vi "oldECG AF SPI Input.vi"() -> ()   [LabVIEW 2013]
uses:
  ECG Data.ctl
  IBP Data.ctl
  Trigger Params.ctl
  Lead Enum.ctl
  <vilib>/Platform/TimedLoop/XDataNode/timing_clust.ctl
  <vilib>/Platform/TimedLoop/XDataNode/nitl_modes.ctl
  <vilib>/Platform/TimedLoop/XDataNode/wakeup.ctl
  Gradient Data.ctl
  All Data.ctl
  <vilib>/rvi/Emulation/niFpgaSctlEmulationGetInTimedLoop.vi
  <vilib>/rvi/Emulation/niFpgaEmulationReportErrorSimple.vi
  <vilib>/rvi/Emulation/niFpgaGetClockAttributes.vi
  <vilib>/rvi/Emulation/niFpgaCriticalErrorInLSC.vi
  <vilib>/rvi/eio/common/nirviEmuTemplateMethod_errors.vi
  <vilib>/rvi/DataTransferAndStorage/Container/Common/niFpgaContainerGetUniqueNameForEmu.vi
  <vilib>/rvi/DataTransferAndStorage/Container/Common/niFpgaContainerSetEmuInfo.vi
  <vilib>/rvi/eio/common/nirviEmuReportErrorAndStop.vi
  <vilib>/rvi/Emulation/niFpgaProcessEmulError.vi
  <vilib>/rvi/Analysis/common/codeGenErrors/XNode/niFpgaXNodeCodeGenErrorHandle.vi
  <vilib>/rvi/DataTransferAndStorage/Container/Common/niFpgaContainerExecOnDevCompGetState.vi
  <vilib>/rvi/FIFO/Fifo_Resource/nirvififoEmulationWriteFpgaImpl.vi
  <vilib>/rvi/interface/RandomDataEmulation/nirviRandomDataFPGAFIFO.vi
  <vilib>/rvi/interface/RandomDataEmulation/niFpgaRandomDataHandleErrors.vi
  <vilib>/rvi/FIFO/Fifo_Resource/nirvififoEmulationGetNumberOfElementsToReadFpgaImpl.vi
  <vilib>/rvi/FIFO/Fifo_Resource/nirvififoEmulationReadFpgaImpl.vi
  <vilib>/Platform/TimedLoop/XDataNode/XDataNode.xnode
  <vilib>/eio/EIONode/EIONode.xnode
  <vilib>/rvi/LocalResourceManager/LocalResourceManager.xnode
  <vilib>/eio/EIOMethodNode/EIOMethodNode.xnode
  <vilib>/rvi/Analysis/measure/butterworth/XNode/niFpgaButterworthFilter.xnode
  <vilib>/rvi/Analysis/measure/LMRsmpl/XNode/niFPGA Rational Resampler.xnode
  <vilib>/rvi/DataTransferAndStorage/Container/XNode/niFpgaContainer.xnode
  <vilib>/rvi/FIFO/Fifo_Resource/niFpgaFifoEmulationRefIn.vi
  <vilib>/Platform/TimedLoop/XDataNode/XDNodeRunTimeDep.lvlib
panel:
  out "LL Out":i16
  out "LA Out":i16
  out "RA Out":i16
  out "LL In":i16
  out "LA In":i16
  out "RA In":i16
  in  "HPF":bool
  in  "Trigger":T1
  out "IBP Data":T3
  out "ECG Data":T4
  in  "stop":bool
  in  "Reset":bool
  out "Send":bool
  out "WeightSum":fxp<+/-,33,19> format="%.20g"
  out "BetaProduct":fxp<+/-,32,-1> format="%.33g"
  out "Loop Time":u32
  in  "Filter Size":i16
  out "I In":i16
  out "II In":i16
  out "III In":i16
  out "aVR In":i16
  out "aVL In":i16
  out "aVF In":i16
  out "V1 In":i16
  out "V2 In":i16
  out "V3 In":i16
  out "V4 In":i16
  out "V5 In":i16
  out "V6 In":i16
  out "V4 Out":i16
  out "V5 Out":i16
  out "V6 Out":i16
  out "IBP3":i16
  out "IBP2":i16
  out "IBP1":i16
  in  "Start 0":bool
  in  "Filter On":bool=TRUE
  in  "Beta":fxp<+/-,32,-16>
  out "V3 Out":i16
  out "V2 Out":i16
  out "V1 Out":i16
  out "aVF Out":i16
  out "aVL Out":i16
  out "aVR Out":i16
  out "III Out":i16
  out "II Out":i16
  out "I Out":i16
  out "V6":i16
  out "V5":i16
  out "V4":i16
  out "V3":i16
  out "V2":i16
  out "V1":i16
  out "LL":i16
  out "LA":i16
  out "Actual Loop Rate (Ticks)":u32
  out "Late? Latched":bool
  out "RA":i16
  in  "Loop Rate (Ticks)":u32=4000
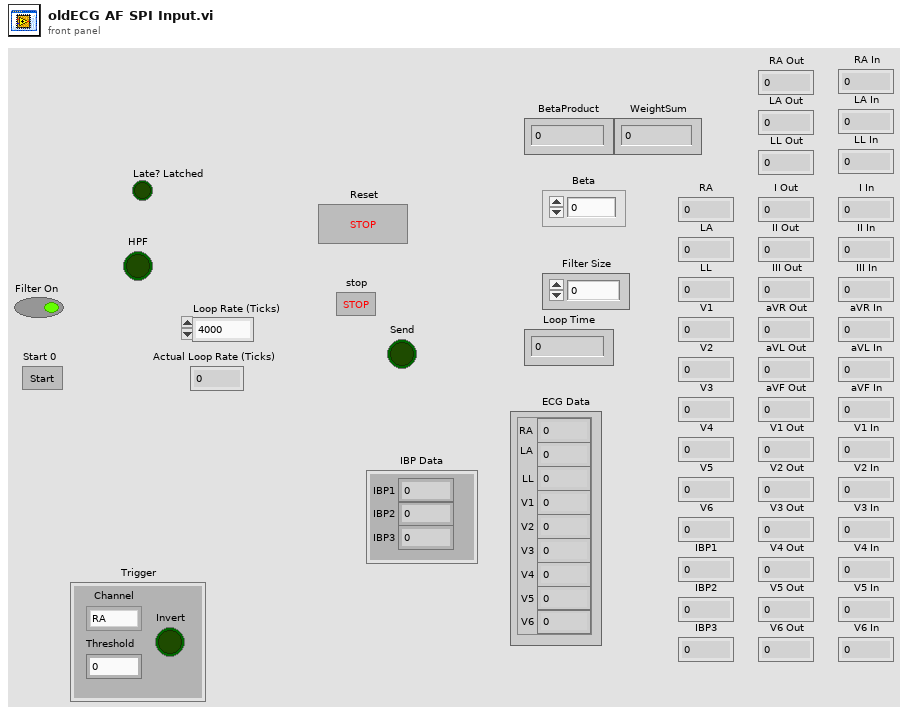
[diagram p1: front panel]
types:
  T1 = typedef "Trigger Params.ctl" = cluster{"Channel":T2, "Threshold":i16, "Invert":bool}
  T2 = typedef "Lead Enum.ctl" = enum16{"RA", "LA", "LL", "V1", "V2", "V3", "V4", "V5", "V6", "I", "II", "III", "aVR", "aVL", "aVF", "Vw"}
  T3 = typedef "IBP Data.ctl" = cluster{"IBP1":fxp<+/-,16,16>, "IBP2":fxp<+/-,16,16>, "IBP3":fxp<+/-,16,16>}
  T4 = typedef "ECG Data.ctl" = cluster{"RA":fxp<+/-,16,16>, "LA":fxp<+/-,16,16>, "LL":fxp<+/-,16,16>, "V1":fxp<+/-,16,16>, "V2":fxp<+/-,16,16>, "V3":fxp<+/-,16,16>, "V4":fxp<+/-,16,16>, "V5":fxp<+/-,16,16>, "V6":fxp<+/-,16,16>}
  T5 = typedef "XDNodeRunTimeDep.lvlib/timing_clust.ctl" = cluster{"Expected End [f-1]":u64, "Actual End [f-1]":u64, "Finished Late? [f-1]":bool, "Expected End [i-1]":u64, "Actual End [i-1]":u64, "Finished Late? [i-1]":bool, "Expected Start [i]":u64, "Actual Start [i]":u64, "Expected Start [f]":u64, "Actual Start [f]":u64, "Source Name":string, "Structure Name":string, "Period":i64, "Deadline":i64, "Offset":i64, "Start":i64, "Priority":i32, "Timeout":i32, "Mode":T6, "Wakeup Reason":T7, "Error":errorcluster, "Source Type":string, "Secondary Source Type":string, "Global End Time":u64, "Global Start Time":u64, "Frame Duration":u64, "Iteration Duration":u64, "Assigned CPU":i32, "I/O Scan Engine Mode":u32}
  T6 = typedef "XDNodeRunTimeDep.lvlib/nitl_modes.ctl" = enum32{"No Change", "Process missed periods, maintain original phase", "Discard missed periods, maintain original phase", "Process missed periods, ignore original phase", "Discard missed periods, ignore original phase"}
  T7 = typedef "XDNodeRunTimeDep.lvlib/wakeup.ctl" = enum32{"Normal", "Aborted", "Asynchronous wakeup", "Timing source error", "Timed loop error", "Timeout"}
  T8 = typedef "Memory Block Channels.ctl" = cluster{"RA":T9, "LA":T9, "LL":T9, "V1":T9, "V2":T9, "V3":T9}
  T9 = typedef "MemoryBlocks.ctl" = cluster{"Taps":refnum<k21>, "Weights":refnum<k21>, "IO Weights":refnum<k21>, "IO Taps":refnum<k21>}
  T10 = cluster{"ECG":cluster{"RA":fxp<+/-,16,16>, "LA":fxp<+/-,16,16>, "LL":fxp<+/-,16,16>, "V1":fxp<+/-,16,16>, "V2":fxp<+/-,16,16>, "V3":fxp<+/-,16,16>, "V4":fxp<+/-,16,16>, "V5":fxp<+/-,16,16>, "V6":fxp<+/-,16,16>}, "Gradients":cluster{"X":fxp<+/-,16,16>, "Y":fxp<+/-,16,16>, "Z":fxp<+/-,16,16>}, "IBP":cluster{"IBP1":fxp<+/-,16,16>, "IBP2":fxp<+/-,16,16>, "IBP3":fxp<+/-,16,16>}}
  T11 = cluster{"BetaProduct":fxp<+/-,32,-1>, "WeightSum":fxp<+/-,33,19>}
  T12 = typedef "ECG Leads.ctl" = cluster{"RA":i16, "LA":i16, "LL":i16, "V1":i16, "V2":i16, "V3":i16, "V4":i16, "V5":i16, "V6":i16, "I":i16, "II":i16, "III":i16, "aVR":i16, "aVL":i16, "aVF":i16, "Vw":i16}
  T13 = cluster{"X":fxp<+/-,16,16>, "Y":fxp<+/-,16,16>, "Z":fxp<+/-,16,16>}
  T14 = cluster{"IBP1":fxp<+/-,16,16>, "IBP2":fxp<+/-,16,16>, "IBP3":fxp<+/-,16,16>}
  T15 = typedef "All Data.ctl" = cluster{"ECG":T4, "Gradients":T16, "IBP":T3}
  T16 = typedef "Gradient Data.ctl" = cluster{"X":fxp<+/-,16,16>, "Y":fxp<+/-,16,16>, "Z":fxp<+/-,16,16>}
  T17 = cluster{"[0]":fxp<+/-,16,16>, "[1]":fxp<+/-,16,16>, "[2]":fxp<+/-,16,16>}
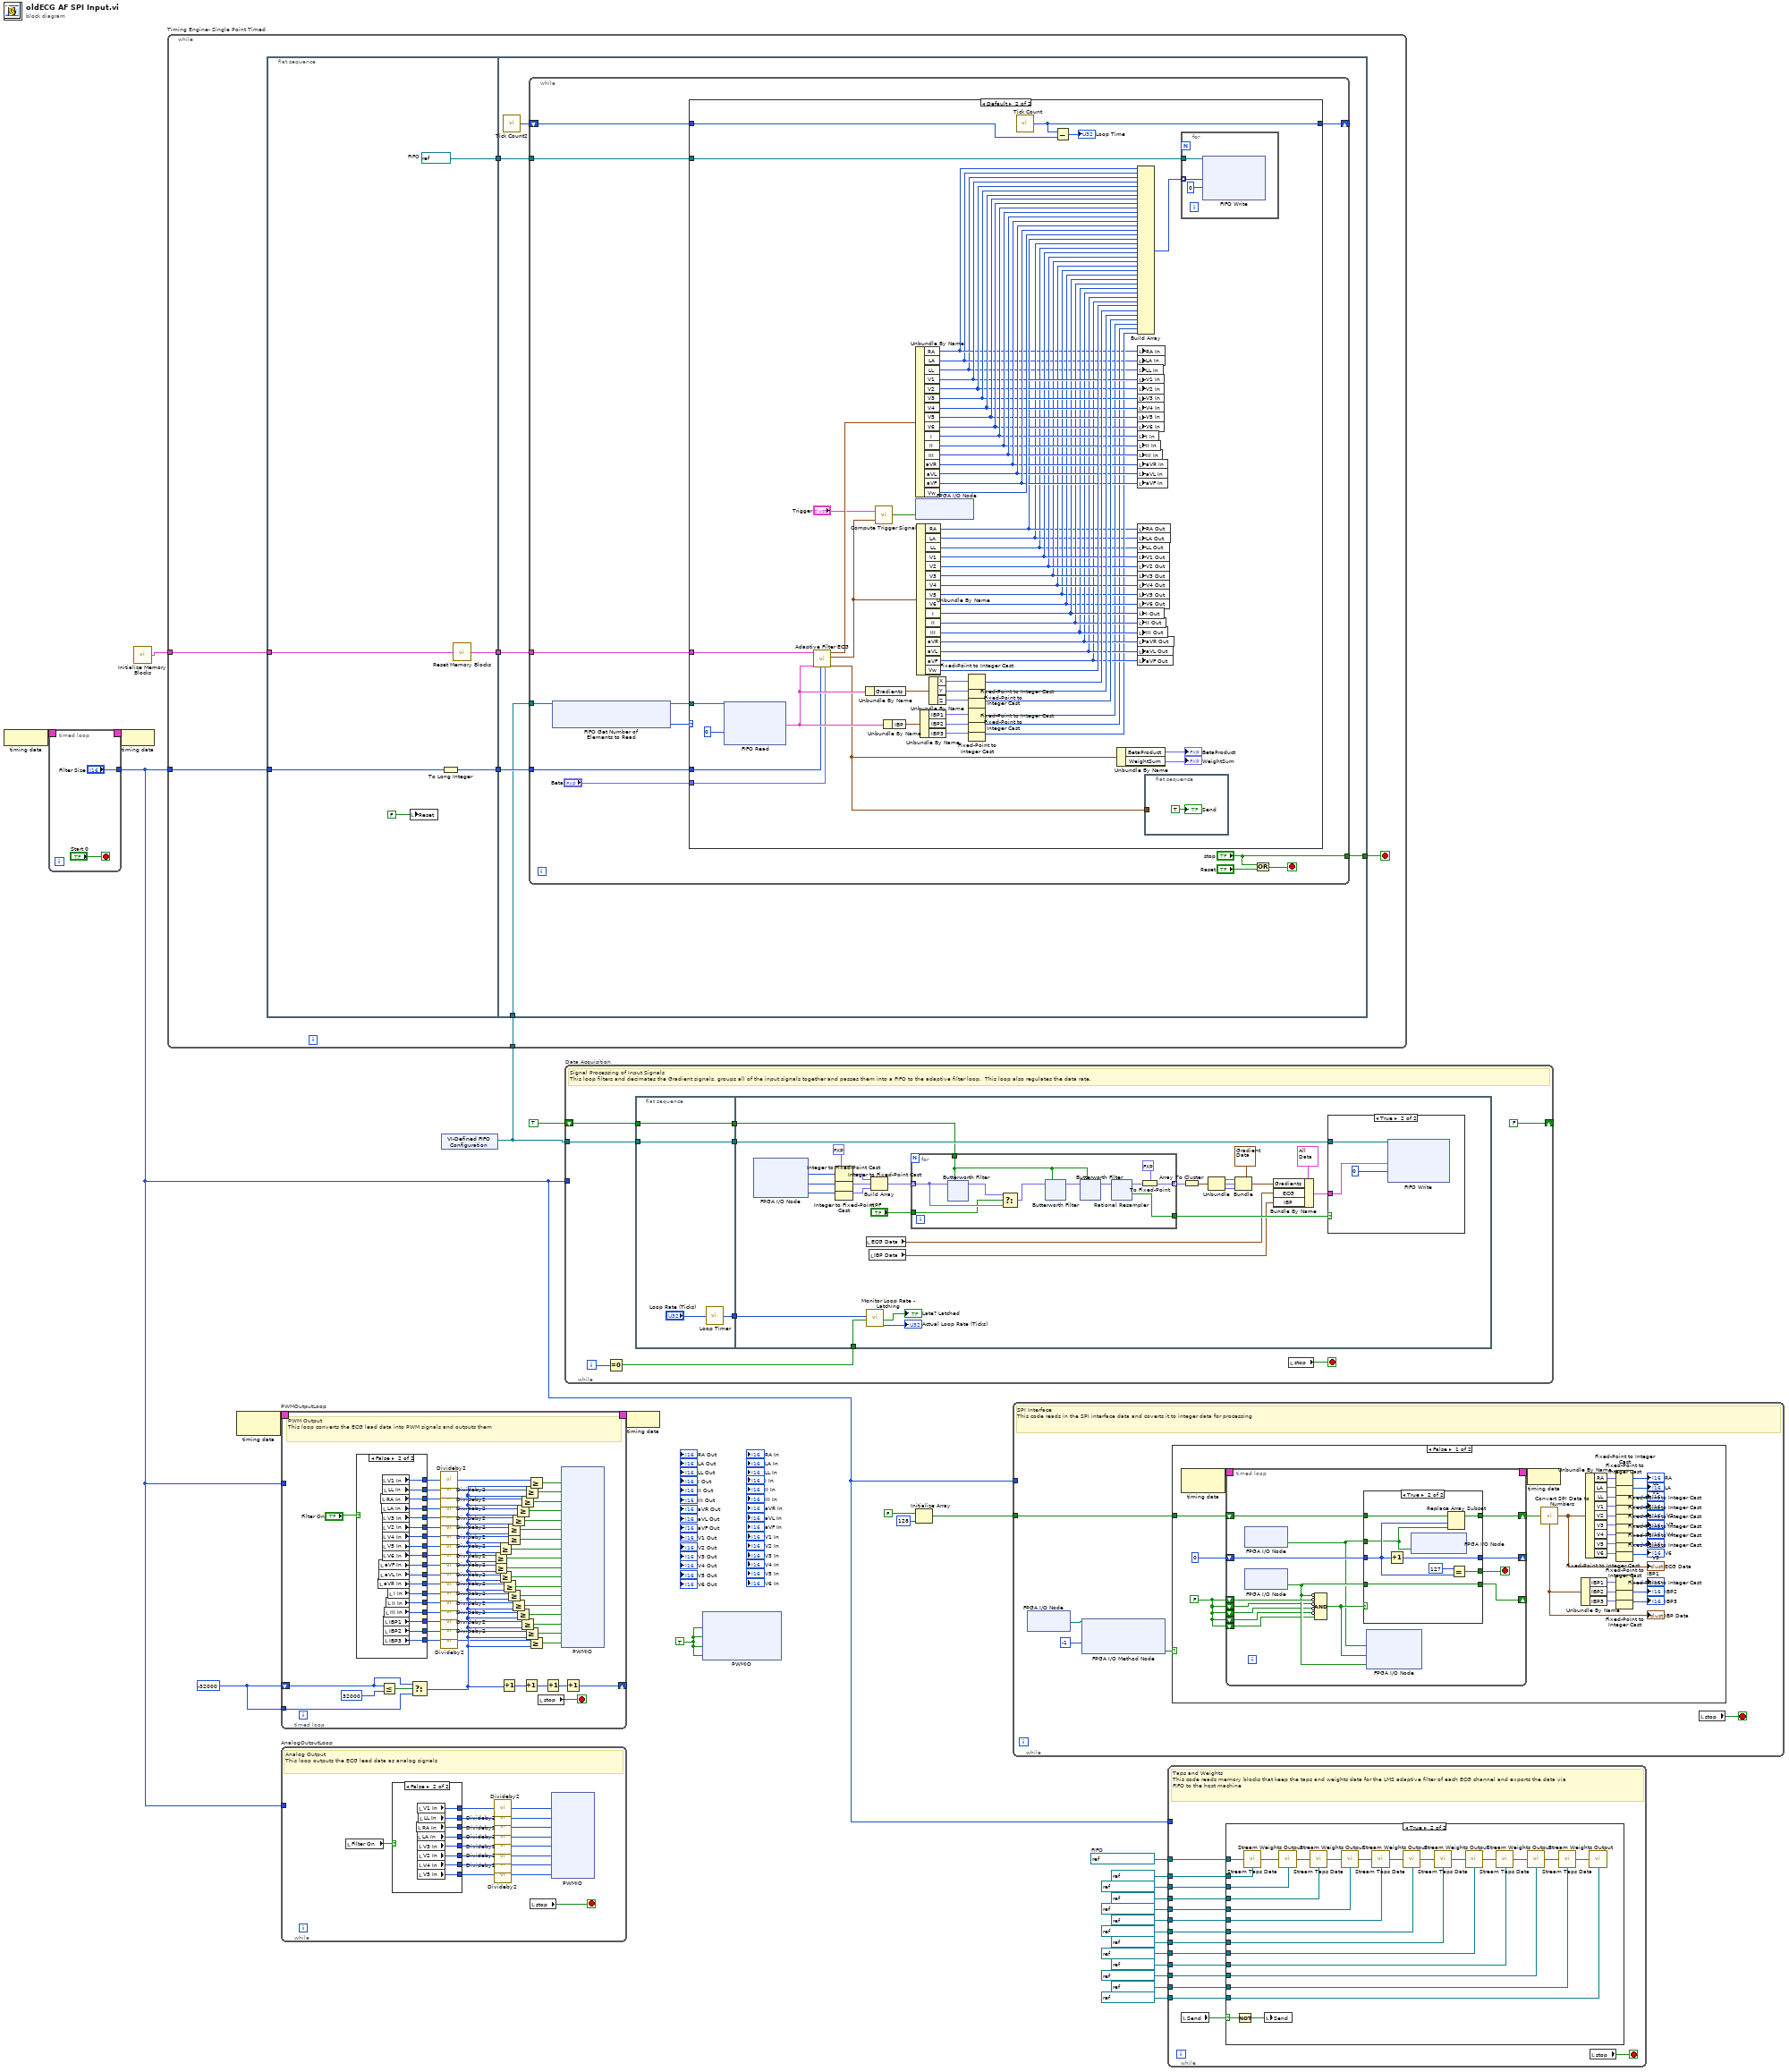
[diagram p0: block diagram]
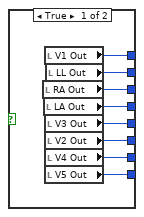
[diagram p4: hidden frame]
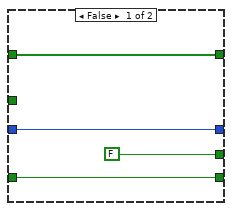
[diagram p5: hidden frame]
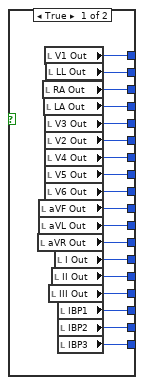
[diagram p7: hidden frame]
diagram:
  w1 = TRUE
  w8 = refnum<k21> "FIFO Filter Specs"  # FIFO
  w24 = i16 -32000
  n1 = node-c288 ("Input Node")() -> (w5:T5)
  n2 = timed-loop "initWait" {
    timing: w5 -> [_]
    timing-out: [_] -> w4
    tunnel: ["Filter Size"] -> w3
    stop <- "Start 0" stop-if-true
  }
  n3 = node-c288 ("Output Node")(w4) -> ()
  n4 = call "Initialize Memory Blocks.vi"() -> ("Memory"=w7:T8)
  n5 = node-c288 ("Input Node")() -> (w26:T5)  [unwired: 1 in]
  n6 = timed-loop "PWMOutputLoop" {
    timing: w26 -> [_]
    timing-out: [_] -> w25
    shift-right: [w76] -> _
    shift-left: w24 -> [w93]
    tunnel: w24 -> [w81]
    tunnel: w3 -> [_]
    stop <- w50 stop-if-true
    # "PWM Output\nThis loop converts the ECG lead data into PWM signals and outputs them"
    n7 = case shown="False" "Filter On" {
      tunnel: [w113 w131] -> w79
      tunnel: [w112 w130] -> w78
      tunnel: [w111 w129] -> w72
      tunnel: [w110 w128] -> w73
      tunnel: [w109 w127] -> w69
      tunnel: [w108 w126] -> w68
      tunnel: [w107 w125] -> w70
      tunnel: [w106 w124] -> w71
      tunnel: [w105 w123] -> w67
      tunnel: [w104 w122] -> w59
      tunnel: [w103 w121] -> w58
      tunnel: [w102 w120] -> w57
      tunnel: [w101 w119] -> w49
      tunnel: [w100 w118] -> w48
      tunnel: [w99 w117] -> w47
      tunnel: [w98 w116] -> w46
      tunnel: [w97 w115] -> w45
      tunnel: [w96 w114] -> w44
      frame True {
        n8 = local read "aVR Out"() -> (w102:i16)
        n9 = local read "aVF Out"() -> (w104:i16)
        n10 = local read "aVL Out"() -> (w103:i16)
        n11 = local read "RA Out"() -> (w110:i16)
        n12 = local read "LA Out"() -> (w111:i16)
        n13 = local read "V1 Out"() -> (w113:i16)
        n14 = local read "V3 Out"() -> (w106:i16)
        n15 = local read "V2 Out"() -> (w107:i16)
        n16 = local read "V4 Out"() -> (w109:i16)
        n17 = local read "V5 Out"() -> (w108:i16)
        n18 = local read "V6 Out"() -> (w105:i16)
        n19 = local read "LL Out"() -> (w112:i16)
        n20 = local read "III Out"() -> (w99:i16)
        n21 = local read "II Out"() -> (w100:i16)
        n22 = local read "I Out"() -> (w101:i16)
        n23 = local read "IBP1"() -> (w98:i16)
        n24 = local read "IBP2"() -> (w97:i16)
        n25 = local read "IBP3"() -> (w96:i16)
      }
      frame False {
        n26 = local read "aVR In"() -> (w120:i16)
        n27 = local read "aVF In"() -> (w122:i16)
        n28 = local read "aVL In"() -> (w121:i16)
        n29 = local read "RA In"() -> (w128:i16)
        n30 = local read "LA In"() -> (w129:i16)
        n31 = local read "V1 In"() -> (w131:i16)
        n32 = local read "V3 In"() -> (w124:i16)
        n33 = local read "V2 In"() -> (w125:i16)
        n34 = local read "V4 In"() -> (w127:i16)
        n35 = local read "V5 In"() -> (w126:i16)
        n36 = local read "V6 In"() -> (w123:i16)
        n37 = local read "LL In"() -> (w130:i16)
        n38 = local read "IBP1"() -> (w116:i16)
        n39 = local read "IBP2"() -> (w115:i16)
        n40 = local read "IBP3"() -> (w114:i16)
        n41 = local read "III In"() -> (w117:i16)
        n42 = local read "II In"() -> (w118:i16)
        n43 = local read "I In"() -> (w119:i16)
      }
    }
    n44 = Less Or Equal?(x=w93, y=i16 32000 ("Period")) -> (x <= y?=w94:bool)
    n45 = Select(t=w93, s=w94, f=w81) -> (s? t:f=w37:i16)
    n46 = call "Divideby2.vi"("Input"=w79) -> ("Output"=w75:i16)
    n47 = call "Divideby2.vi"("Input"=w78) -> ("Output"=w74:i16)
    n48 = call "Divideby2.vi"("Input"=w73) -> ("Output"=w60:i16)
    n49 = call "Divideby2.vi"("Input"=w72) -> ("Output"=w61:i16)
    n50 = call "Divideby2.vi"("Input"=w71) -> ("Output"=w62:i16)
    n51 = call "Divideby2.vi"("Input"=w70) -> ("Output"=w63:i16)
    n52 = call "Divideby2.vi"("Input"=w69) -> ("Output"=w64:i16)
    n53 = call "Divideby2.vi"("Input"=w68) -> ("Output"=w65:i16)
    n54 = call "Divideby2.vi"("Input"=w67) -> ("Output"=w66:i16)
    n55 = call "Divideby2.vi"("Input"=w59) -> ("Output"=w56:i16)
    n56 = call "Divideby2.vi"("Input"=w58) -> ("Output"=w55:i16)
    n57 = call "Divideby2.vi"("Input"=w57) -> ("Output"=w54:i16)
    n58 = call "Divideby2.vi"("Input"=w49) -> ("Output"=w32:i16)
    n59 = call "Divideby2.vi"("Input"=w48) -> ("Output"=w33:i16)
    n60 = call "Divideby2.vi"("Input"=w47) -> ("Output"=w31:i16)
    n61 = call "Divideby2.vi"("Input"=w46) -> ("Output"=w34:i16)
    n62 = call "Divideby2.vi"("Input"=w45) -> ("Output"=w35:i16)
    n63 = call "Divideby2.vi"("Input"=w44) -> ("Output"=w36:i16)
    n64 = Greater Or Equal?(x=w66, y=w37) -> (x >= y?=w83:bool)
    n65 = Greater Or Equal?(x=w56, y=w37) -> (x >= y?=w53:bool)
    n66 = Greater Or Equal?(x=w65, y=w37) -> (x >= y?=w84:bool)
    n67 = Greater Or Equal?(x=w55, y=w37) -> (x >= y?=w52:bool)
    n68 = Increment(x=w37) -> (x+1=w92:i16)
    n69 = Greater Or Equal?(x=w54, y=w37) -> (x >= y?=w51:bool)
    n70 = Greater Or Equal?(x=w63, y=w37) -> (x >= y?=w86:bool)
    n71 = Greater Or Equal?(x=w64, y=w37) -> (x >= y?=w85:bool)
    n72 = Greater Or Equal?(x=w32, y=w37) -> (x >= y?=w38:bool)
    n73 = Greater Or Equal?(x=w62, y=w37) -> (x >= y?=w87:bool)
    n74 = Greater Or Equal?(x=w33, y=w37) -> (x >= y?=w39:bool)
    n75 = Greater Or Equal?(x=w61, y=w37) -> (x >= y?=w88:bool)
    n76 = Greater Or Equal?(x=w31, y=w37) -> (x >= y?=w40:bool)
    n77 = Greater Or Equal?(x=w60, y=w37) -> (x >= y?=w89:bool)
    n78 = Greater Or Equal?(x=w34, y=w37) -> (x >= y?=w41:bool)
    n79 = Increment(x=w92) -> (x+1=w80:i16)
    n80 = Greater Or Equal?(x=w74, y=w37) -> (x >= y?=w90:bool)
    n81 = Greater Or Equal?(x=w35, y=w37) -> (x >= y?=w42:bool)
    n82 = Greater Or Equal?(x=w75, y=w37) -> (x >= y?=w91:bool)
    n83 = Greater Or Equal?(x=w36, y=w37) -> (x >= y?=w43:bool)
    n84 = local read "stop"() -> (w50:bool)
    n85 = Increment(x=w80) -> (x+1=w77:i16)
    n86 = xnode ("PWMIO")("V1"=w91, "LL"=w90, "RA"=w89, "LA"=w88, "V3"=w87, "V2"=w86, "V4"=w85, "V5"=w84, "V6"=w83, "aVF"=w53, "aVL"=w52, "aVR"=w51, "I"=w38, "II"=w39, "III"=w40, "IBP1"=w41, "IBP2"=w42, "IBP3"=w43) -> ()  [unwired: 18 in, 18 out]
    n87 = Increment(x=w77) -> (x+1=w76:i16)
  }
  n88 = while "AnalogOutputLoop" {
    tunnel: w3 -> [_]
    stop <- w134 stop-if-true
    # "Analog Output\nThis loop outputs the ECG lead data as analog signals"
    n89 = local read "Filter On"() -> (w151:bool)
    n90 = case shown="False" w151 {
      tunnel: [w159 w167] -> w150
      tunnel: [w158 w166] -> w149
      tunnel: [w157 w165] -> w147
      tunnel: [w156 w164] -> w148
      tunnel: [w155 w163] -> w144
      tunnel: [w154 w162] -> w143
      tunnel: [w153 w161] -> w145
      tunnel: [w152 w160] -> w146
      frame True {
        n91 = local read "RA Out"() -> (w156:i16)
        n92 = local read "LA Out"() -> (w157:i16)
        n93 = local read "V1 Out"() -> (w159:i16)
        n94 = local read "V3 Out"() -> (w152:i16)
        n95 = local read "V2 Out"() -> (w153:i16)
        n96 = local read "V4 Out"() -> (w155:i16)
        n97 = local read "V5 Out"() -> (w154:i16)
        n98 = local read "LL Out"() -> (w158:i16)
      }
      frame False {
        n99 = local read "RA In"() -> (w164:i16)
        n100 = local read "LA In"() -> (w165:i16)
        n101 = local read "V1 In"() -> (w167:i16)
        n102 = local read "V3 In"() -> (w160:i16)
        n103 = local read "V2 In"() -> (w161:i16)
        n104 = local read "V4 In"() -> (w163:i16)
        n105 = local read "V5 In"() -> (w162:i16)
        n106 = local read "LL In"() -> (w166:i16)
      }
    }
    n107 = call "Divideby2.vi"("Input"=w150) -> ("Output"=w142:i16)
    n108 = call "Divideby2.vi"("Input"=w149) -> ("Output"=w141:i16)
    n109 = call "Divideby2.vi"("Input"=w148) -> ("Output"=w140:i16)
    n110 = call "Divideby2.vi"("Input"=w147) -> ("Output"=w139:i16)
    n111 = call "Divideby2.vi"("Input"=w146) -> ("Output"=w138:i16)
    n112 = call "Divideby2.vi"("Input"=w145) -> ("Output"=w137:i16)
    n113 = call "Divideby2.vi"("Input"=w144) -> ("Output"=w136:i16)
    n114 = call "Divideby2.vi"("Input"=w143) -> ("Output"=w135:i16)
    n115 = local read "stop"() -> (w134:bool)
    n116 = xnode ("PWMIO")("ECG0"=w142, "ECG1"=w141, "ECG2"=w140, "ECG3"=w139, "ECG4"=w138, "ECG5"=w137, "ECG6"=w136, "ECG7"=w135) -> ()  [unwired: 8 in, 8 out]
  }
  n117 = xnode "VI-Defined FIFO Configuration"() -> ("FIFO Out"=w6:refnum<k21>)
  n118 = while "Timing Engine- Single Point Timed" {
    tunnel: w7 -> [w170]
    tunnel: w6 -> [w169]
    tunnel: w3 -> [w168]
    stop <- w171 stop-if-true
    n119 = flat-sequence "MainSeq" {
      tunnel: [w180] -> w174
      tunnel: [w179] -> w173
      tunnel: [w178] -> w172
      tunnel: w170 -> [w177]
      tunnel: w168 -> [w176]
      tunnel: w174 -> [w186]
      tunnel: w173 -> [w185]
      tunnel: w172 -> [w184]
      tunnel: [w182] -> w171
      tunnel: w169 -> [w181]
      frame #0 {
        w180 = refnum<k21> "FIFO"  # FIFO
        n120 = local write "Reset"(FALSE ("Reset")) -> ()
        n121 = To Long Integer(number=w176) -> (32bit integer=w179:i32)
        n122 = call "Reset Memory Blocks.vi"("Memory Blocks In"=w177) -> ("Memory Blocks Out"=w178:T8)  [unwired: 1 in]
      }
      frame #1 {
        n123 = call "Tick Count2"() -> ("Tick Count(uSec)"=w183:u32)
        n124 = while {
          tunnel: w181 -> [w198]
          tunnel: w186 -> [w194]
          tunnel: w185 -> [w193]
          tunnel: w184 -> [w187]
          shift-right: [w192] -> _
          shift-left: w183 -> [w191]
          tunnel: ["stop"] -> w182
          stop <- w189 stop-if-true
          n125 = xnode ("FIFO Get Number of Elements to Read")("FIFO In"=w198) -> ("Number of Elements to Read"=w197:u32, "FIFO Out"=w196:refnum<k21>)
          n126 = case shown="Default" w197 {
            tunnel: w196 -> [_ w263]
            tunnel: "Beta" -> [_ w209]
            tunnel: w194 -> [_ w261]
            tunnel: w193 -> [_ w210]
            tunnel: w191 -> [w199 w224]
            tunnel: [w199 w225] -> w192
            tunnel: w187 -> [_ w221]
            frame 0 {
            }
            frame Default {
              n127 = xnode ("FIFO Read")("Timeout"=0, "FIFO In"=w263) -> ("Element"=w212:T10)  [unwired: 2 out]
              n128 = call "Adaptive Filter ECG.vi"("Beta"=w209, "Filter Length"=w210, "Data in"=w212, "Memory Blocks In"=w221) -> ("Data"=w211:T11, "Filtered Leads"=w208:T12, "Raw Leads"=w256:T12)  [unwired: 5 in]
              n129 = Unbundle By Name(w212) -> ("Gradients"=w220:T13)
              n130 = call "Compute Trigger Signal.vi"("Leads"=w208, "Trigger"="Trigger") -> ("Trigger Out"=w206:bool)
              n131 = Unbundle By Name(w212) -> ("IBP"=w217:T14)
              n132 = xnode "FPGA I/O Node"("Trigger Out"=w206) -> ()  [unwired: 1 in, 1 out]
              n133 = Unbundle By Name(w256) -> ("RA"=w202:i16, "LA"=w201:i16, "LL"=w200:i16, "V1"=w239:i16, "V2"=w240:i16, "V3"=w241:i16, "V4"=w242:i16, "V5"=w243:i16, "V6"=w244:i16, "I"=w245:i16, "II"=w246:i16, "III"=w247:i16, "aVR"=w248:i16, "aVL"=w249:i16, "aVF"=w250:i16, "Vw"=w255:i16)
              n134 = Unbundle By Name(w208) -> ("RA"=w205:i16, "LA"=w204:i16, "LL"=w203:i16, "V1"=w238:i16, "V2"=w237:i16, "V3"=w236:i16, "V4"=w235:i16, "V5"=w227:i16, "V6"=w228:i16, "I"=w234:i16, "II"=w233:i16, "III"=w232:i16, "aVR"=w231:i16, "aVL"=w230:i16, "aVF"=w229:i16, "Vw"=w254:i16)
              n135 = Unbundle By Name(w217) -> ("IBP1"=w216:fxp<+/-,16,16>, "IBP2"=w215:fxp<+/-,16,16>, "IBP3"=w214:fxp<+/-,16,16>)
              n136 = Unbundle By Name(w220) -> ("X"=w259:fxp<+/-,16,16>, "Y"=w258:fxp<+/-,16,16>, "Z"=w257:fxp<+/-,16,16>)
              n137 = Fixed-Point to Integer Cast(1:w259) -> (0:w253:i16)
              n138 = Fixed-Point to Integer Cast(1:w258) -> (0:w252:i16)
              n139 = Fixed-Point to Integer Cast(1:w257) -> (0:w251:i16)
              n140 = Fixed-Point to Integer Cast(1:w216) -> (0:w219:i16)
              n141 = Fixed-Point to Integer Cast(1:w215) -> (0:w218:i16)
              n142 = Fixed-Point to Integer Cast(1:w214) -> (0:w213:i16)
              n143 = call "Tick Count"() -> ("Tick Count(uSec)"=w225:u32)
              n144 = Subtract(x=w225, y=w224) -> (x-y=→"Loop Time":u32)
              n145 = Unbundle By Name(w211) -> ("BetaProduct"=→"BetaProduct":fxp<+/-,32,-1>, "WeightSum"=→"WeightSum":fxp<+/-,33,19>)
              n146 = Build Array(w202, w201, w200, w239, w240, w241, w242, w243, w244, w245, w246, w247, w248, w249, w250, w255, w205, w204, w203, w238, w237, w236, w235, w227, w228, w234, w233, w232, w231, w230, w229, w254, w253, w252, w251, w219, w218, w213) -> (w260:i16[])
              n147 = local write "RA In"(w202) -> ()
              n148 = local write "LA In"(w201) -> ()
              n149 = local write "LL In"(w200) -> ()
              n150 = local write "V1 In"(w239) -> ()
              n151 = local write "V2 In"(w240) -> ()
              n152 = local write "V3 In"(w241) -> ()
              n153 = local write "V4 In"(w242) -> ()
              n154 = local write "V5 In"(w243) -> ()
              n155 = local write "V6 In"(w244) -> ()
              n156 = local write "I In"(w245) -> ()
              n157 = local write "II In"(w246) -> ()
              n158 = local write "III In"(w247) -> ()
              n159 = local write "aVR In"(w248) -> ()
              n160 = local write "aVL In"(w249) -> ()
              n161 = local write "aVF In"(w250) -> ()
              n162 = local write "RA Out"(w205) -> ()
              n163 = local write "LA Out"(w204) -> ()
              n164 = local write "LL Out"(w203) -> ()
              n165 = local write "V1 Out"(w238) -> ()
              n166 = local write "V2 Out"(w237) -> ()
              n167 = local write "V3 Out"(w236) -> ()
              n168 = local write "V4 Out"(w235) -> ()
              n169 = local write "V5 Out"(w227) -> ()
              n170 = local write "V6 Out"(w228) -> ()
              n171 = local write "I Out"(w234) -> ()
              n172 = local write "II Out"(w233) -> ()
              n173 = local write "III Out"(w232) -> ()
              n174 = local write "aVR Out"(w231) -> ()
              n175 = local write "aVL Out"(w230) -> ()
              n176 = local write "aVF Out"(w229) -> ()
              n177 = flat-sequence {
                tunnel: w211 -> [_]
                frame #0 {
                  "Send" <- TRUE ("Send")
                }
              }
              n178 = for {
                tunnel: w261 -> [w267]
                tunnel: w260 -> [w265] mode=indexing
                n179 = xnode ("FIFO Write")("Element"=w265, "Timeout"=0, "FIFO In"=w267) -> ()  [unwired: 2 out]
              }
            }
          }
          n180 = Or(x="stop", y="Reset") -> (x .or. y?=w189:bool)
        }
      }
    }
  }
  n181 = while "Data Acquisition" {
    tunnel: w6 -> [w275]
    tunnel: w3 -> [_]
    shift-right: [FALSE] -> _
    shift-left: TRUE -> [w270]
    i -> [w273]
    stop <- w271 stop-if-true
    # "Signal Processing of Input Signals\nThis loop filters and decimates the Gradient signals, groups all of the input signals together and passes them into a FIFO to the adaptive filter loop.  This loop also regulates the data rate."
    n182 = Equal To 0?(x=w273) -> (x = 0?=w272:bool)
    n183 = flat-sequence "Data Acquisition Sequence" {
      tunnel: ["Loop Rate (Ticks)"] -> w276
      tunnel: w275 -> [w279]
      tunnel: [w279] -> w274
      tunnel: w270 -> [w277]
      tunnel: [w277] -> w269
      tunnel: w276 -> [w304]
      tunnel: w272 -> [w305]
      tunnel: w274 -> [w303]
      tunnel: w269 -> [w281]
      frame #0 {
        n184 = call "Loop Timer"("Count(Ticks)"="Loop Rate (Ticks)") -> ()  [unwired: 1 out]
      }
      frame #1 {
        w293 = fxp<+/-,16,16> 0.0 ("fixed-point type")
        n185 = xnode "FPGA I/O Node"() -> ("X Gradient"=w296:i16, "Y Gradient"=w295:i16, "Z Gradient"=w294:i16)  [unwired: 3 in, 3 out]
        n186 = Integer to Fixed-Point Cast(fixed-point type=w293, integer=w296) -> (fixed-point=w298:fxp<+/-,16,16>)
        n187 = Integer to Fixed-Point Cast(fixed-point type=w293, integer=w295) -> (fixed-point=w299:fxp<+/-,16,16>)
        n188 = Integer to Fixed-Point Cast(fixed-point type=w293, integer=w294) -> (fixed-point=w297:fxp<+/-,16,16>)
        n189 = local read "ECG Data"() -> (w283:T4)
        n190 = call "Monitor Loop Rate - Latching.vi"("Reset"=w305, "Count(Ticks)"=w304) -> ("Actual Loop Rate (Ticks)"=→"Actual Loop Rate (Ticks)":u32, "Late? (Latched)"=→"Late? Latched":bool)  [unwired: 7 in, 1 out]
        n191 = local read "IBP Data"() -> (w282:T3)
        n192 = Build Array(w298, w299, w297) -> (w300:fxp<+/-,16,16>[])
        n193 = for {
          tunnel: w300 -> [w309] mode=indexing
          tunnel: [w313] -> w292 mode=indexing
          tunnel: [w314] -> w302
          tunnel: w281 -> [w311]
          tunnel: "HPF" -> [w307]
          n194 = xnode "Butterworth Filter"("input data"=w309, "reset"=w311) -> ("output data"=w310:fxp<+/-,16,16>)  [unwired: 1 in, 1 out]
          n195 = Select(t=w310, s=w307, f=w309) -> (s? t:f=w308:fxp<+/-,16,16>)
          n196 = xnode "Butterworth Filter"("input data"=w308, "reset"=w311) -> ("output data"=w317:fxp<+/-,16,16>)  [unwired: 1 in, 1 out]
          n197 = xnode "Butterworth Filter"("input data"=w317, "reset"=w311) -> ("output data"=w316:fxp<+/-,16,16>)  [unwired: 1 in, 1 out]
          n198 = xnode "Rational Resampler"("input data"=w316) -> ("output data"=w315:fxp<+/-,18,16>, "output valid"=w314:bool)  [unwired: 1 out]
          n199 = To Fixed-Point(fixed-point type=fxp<+/-,16,16> 0.0, number=w315) -> (fixed-point=w313:fxp<+/-,16,16>)
        }
        n200 = Array To Cluster(array=w292) -> (cluster=w291:T17)
        n201 = Unbundle(w291) -> ("[0]"=w289:fxp<+/-,16,16>, "[1]"=w288:fxp<+/-,16,16>, "[2]"=w287:fxp<+/-,16,16>)
        n202 = Bundle(cluster=T16 {"X"=0.0, "Y"=0.0, "Z"=0.0} ("Gradients"), "X"=w289, "Y"=w288, "Z"=w287) -> (w285:T16)
        n203 = Bundle By Name(cluster=T15 {"ECG"={"RA"=0.0, "LA"=0.0, "LL"=0.0, "V1"=0.0, "V2"=0.0, "V3"=0.0, "V4"=0.0, "V5"=0.0, "V6"=0.0}, "Gradients"={"X"=0.0, "Y"=0.0, "Z"=0.0}, "IBP"={"IBP1"=0.0, "IBP2"=0.0, "IBP3"=0.0}} ("Data"), "Gradients"=w285, "ECG"=w283, "IBP"=w282) -> (w284:T15)
        n204 = case shown="True" w302 {
          tunnel: w303 -> [_ w397]
          tunnel: w284 -> [_ w395]
          frame False {
          }
          frame True {
            n205 = xnode ("FIFO Write")("Element"=w395, "Timeout"=0, "FIFO In"=w397) -> ()  [unwired: 2 out]
          }
        }
      }
    }
    n206 = local read "stop"() -> (w271:bool)
  }
  n207 = node-c288 ("Output Node")(w25) -> ()
  n208 = xnode ("PWMIO")("Connector0/DIO19"=w1, "Connector0/DIO20"=w1, "Connector0/DIO21"=w1, "Connector0/DIO22"=w1) -> ()  [unwired: 4 in, 4 out]
  n209 = Initialize Array(FALSE, 128 ("dimension size")) -> (w23:bool[])
  n210 = while {
    tunnel: w23 -> [w399]
    tunnel: w3 -> [_]
    stop <- w398 stop-if-true
    # "SPI Interface\nThis code reads in the SPI interface data and coverts it to integer data for processing"
    n211 = xnode "FPGA I/O Node"() -> ("FPGA I/O Out"=w400:refnum<k21>)  [unwired: 1 in, 1 out]
    n212 = xnode "FPGA I/O Method Node"("FPGA I/O In"=w400, "Timeout"=-1) -> ("Timed Out"=w401:bool)  [unwired: 1 out]
    n213 = case shown="False" w401 {
      tunnel: w399 -> [w434 _]
      frame False {
        w430 = FALSE
        n214 = node-c288() -> (w433:T5)  [unwired: 1 in]
        n215 = timed-loop {
          shift-right: [w446] -> w429
          shift-left: w434 -> [w447]
          timing: w433 -> [_]
          timing-out: [_] -> w432
          shift-right: [w442] -> _
          shift-left: w430 -> [w445]
          shift-right: [w443] -> _
          shift-left: u8 0 -> [w444]
          shift-left: w430 -> [w438]
          shift-left: w430 -> [w437]
          shift-left: w430 -> [w436]
          shift-left: w430 -> [w435]
          stop <- w448 stop-if-true
          n216 = xnode "FPGA I/O Node"() -> ("MOSI"=w439:bool)  [unwired: 1 in, 1 out]
          n217 = xnode "FPGA I/O Node"() -> ("SCLK"=w441:bool)  [unwired: 1 in, 1 out]
          n218 = Compound Arithmetic op=AND(invert w441, invert w445, invert w438, invert w437, invert w436, w435) -> (w440:bool)
          n219 = case shown="True" w440 {
            tunnel: [FALSE w459] -> w448
            tunnel: w447 -> [w449 w458]
            tunnel: [w449 w457] -> w446
            tunnel: w444 -> [w452 w456]
            tunnel: [w452 w455] -> w443
            tunnel: w441 -> [w451 w454]
            tunnel: [w451 w454] -> w442
            tunnel: w439 -> [_ w453]
            frame False {
            }
            frame True {
              n220 = Increment(x=w456) -> (x+1=w455:u8)
              n221 = xnode "FPGA I/O Node"("MOSI Data"=w453) -> ()  [unwired: 1 in, 1 out]
              n222 = Replace Array Subset(array=w458, new element=w453, index=w456) -> (w457:bool[])
              n223 = Equal?(x=u8 127, y=w456) -> (x = y?=w459:bool)
            }
          }
          n224 = xnode "FPGA I/O Node"("MOSI Out"=w439, "SCLK Edge"=w440, "SCLK Out"=w441) -> ()  [unwired: 3 in, 3 out]
        }
        n225 = node-c288(w432) -> ()
        n226 = call "Convert SPI Data to Numbers.vi"("Data In"=w429) -> ("IBP Data"=w409:T3, "ECG Data"=w420:T4)
        "ECG Data" <- w420
        "IBP Data" <- w409
        n227 = Unbundle By Name(w409) -> ("IBP1"=w408:fxp<+/-,16,16>, "IBP2"=w406:fxp<+/-,16,16>, "IBP3"=w404:fxp<+/-,16,16>)
        n228 = Unbundle By Name(w420) -> ("RA"=w428:fxp<+/-,16,16>, "LA"=w427:fxp<+/-,16,16>, "LL"=w426:fxp<+/-,16,16>, "V1"=w425:fxp<+/-,16,16>, "V2"=w424:fxp<+/-,16,16>, "V3"=w423:fxp<+/-,16,16>, "V4"=w422:fxp<+/-,16,16>, "V5"=w421:fxp<+/-,16,16>, "V6"=w411:fxp<+/-,16,16>)
        n229 = Fixed-Point to Integer Cast(1:w428) -> (0:→"RA":i16)
        n230 = Fixed-Point to Integer Cast(1:w427) -> (0:→"LA":i16)
        n231 = Fixed-Point to Integer Cast(1:w426) -> (0:→"LL":i16)
        n232 = Fixed-Point to Integer Cast(1:w425) -> (0:→"V1":i16)
        n233 = Fixed-Point to Integer Cast(1:w424) -> (0:→"V2":i16)
        n234 = Fixed-Point to Integer Cast(1:w423) -> (0:→"V3":i16)
        n235 = Fixed-Point to Integer Cast(1:w422) -> (0:→"V4":i16)
        n236 = Fixed-Point to Integer Cast(1:w421) -> (0:→"V5":i16)
        n237 = Fixed-Point to Integer Cast(1:w411) -> (0:→"V6":i16)
        n238 = Fixed-Point to Integer Cast(1:w408) -> (0:→"IBP1":i16)
        n239 = Fixed-Point to Integer Cast(1:w406) -> (0:→"IBP2":i16)
        n240 = Fixed-Point to Integer Cast(1:w404) -> (0:→"IBP3":i16)
      }
      frame True {
      }
    }
    n241 = local read "stop"() -> (w398:bool)
  }
  n242 = while {
    tunnel: w8 -> [w478]
    tunnel: refnum<k21> "IO Taps 0" ("Memory") -> [w477]
    tunnel: refnum<k21> "IO Weights 0" ("Memory In") -> [w476]
    tunnel: refnum<k21> "IO Taps 1" ("Memory") -> [w475]
    tunnel: refnum<k21> "IO Weights 1" ("Memory In") -> [w474]
    tunnel: refnum<k21> "IO Taps 2" ("Memory") -> [w473]
    tunnel: refnum<k21> "IO Weights 2" ("Memory In") -> [w472]
    tunnel: refnum<k21> "IO Taps 3" ("Memory") -> [w471]
    tunnel: refnum<k21> "IO Weights 3" ("Memory In") -> [w470]
    tunnel: refnum<k21> "IO Taps 4" ("Memory") -> [w469]
    tunnel: refnum<k21> "IO Weights 4" ("Memory In") -> [w468]
    tunnel: refnum<k21> "IO Taps 5" ("Memory") -> [w467]
    tunnel: refnum<k21> "IO Weights 5" ("Memory In") -> [w466]
    tunnel: w3 -> [_]
    stop <- w465 stop-if-true
    # "Taps and Weights\nThis code reads memory blocks that keep the taps and weights data for the LMS adaptive filter of each ECG channel and exports the data via\nFIFO to the host machine"
    n243 = local read "Send"() -> (w479:bool)
    n244 = case shown="True" w479 {
      selector: w479 -> [_ w505]
      tunnel: w478 -> [_ w503]
      tunnel: w477 -> [_ w501]
      tunnel: w476 -> [_ w500]
      tunnel: w475 -> [_ w497]
      tunnel: w474 -> [_ w496]
      tunnel: w473 -> [_ w494]
      tunnel: w472 -> [_ w493]
      tunnel: w471 -> [_ w489]
      tunnel: w470 -> [_ w488]
      tunnel: w469 -> [_ w483]
      tunnel: w468 -> [_ w482]
      tunnel: w467 -> [_ w481]
      tunnel: w466 -> [_ w480]
      frame False {
      }
      frame True {
        n245 = Not(x=w505) -> (.not. x?=w504:bool)
        n246 = call "Stream Taps Data.vi"("FIFO In"=w503, "Memory"=w501) -> ("FIFO out"=w502:refnum<k21>)
        n247 = local write "Send"(w504) -> ()
        n248 = call "Stream Weights Output.vi"("FIFO in"=w502, "Memory In"=w500) -> ("FIFO out"=w498:refnum<k21>)
        n249 = call "Stream Taps Data.vi"("FIFO In"=w498, "Memory"=w497) -> ("FIFO out"=w499:refnum<k21>)
        n250 = call "Stream Weights Output.vi"("FIFO in"=w499, "Memory In"=w496) -> ("FIFO out"=w495:refnum<k21>)
        n251 = call "Stream Taps Data.vi"("FIFO In"=w495, "Memory"=w494) -> ("FIFO out"=w492:refnum<k21>)
        n252 = call "Stream Weights Output.vi"("FIFO in"=w492, "Memory In"=w493) -> ("FIFO out"=w491:refnum<k21>)
        n253 = call "Stream Taps Data.vi"("FIFO In"=w491, "Memory"=w489) -> ("FIFO out"=w490:refnum<k21>)
        n254 = call "Stream Weights Output.vi"("FIFO in"=w490, "Memory In"=w488) -> ("FIFO out"=w484:refnum<k21>)
        n255 = call "Stream Taps Data.vi"("FIFO In"=w484, "Memory"=w483) -> ("FIFO out"=w485:refnum<k21>)
        n256 = call "Stream Weights Output.vi"("FIFO in"=w485, "Memory In"=w482) -> ("FIFO out"=w486:refnum<k21>)
        n257 = call "Stream Taps Data.vi"("FIFO In"=w486, "Memory"=w481) -> ("FIFO out"=w487:refnum<k21>)
        n258 = call "Stream Weights Output.vi"("FIFO in"=w487, "Memory In"=w480) -> ()  [unwired: 1 out]
      }
    }
    n259 = local read "stop"() -> (w465:bool)
  }
